vi "Example Program.vi"() -> ()   [LabVIEW 2014]
uses:
  Type Definitions/UTILITY Power Analyzer.ctl
panel:
  out "Average Power (Watts)":dbl format="%.3f"
  out "Output File":string[][](array[string])
  in  "Power Analyzer":T1
  in  "File Path Control":path=path "C:/Users/220038920/Desktop/CVS Folder/NI-2010/Trunk/Utility/Standby Power/Standby Power Settings.csv"
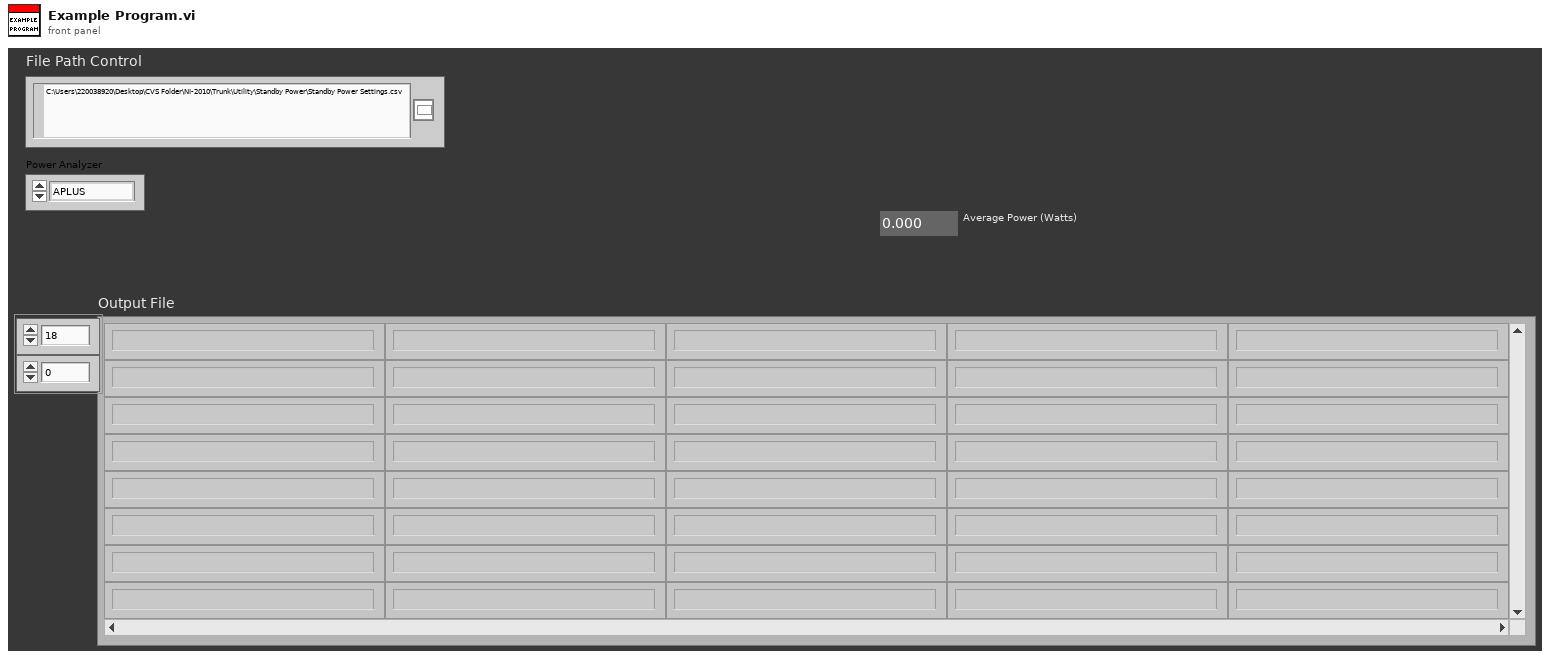
[diagram p1: front panel]
types:
  T1 = typedef "UTILITY Power Analyzer.ctl" = enum16{"APLUS", "WT210", "WT500", "WT300", "OSI", "Debug"}
  T2 = typedef "UTILITY Power Inputs Control.ctl" = cluster{"Yokogawa":cluster{"WT210":cluster{"Sample Rate (1: 0.25s)":i32, "A Range (12: 20A)":i32, "V Range (6: 600V)":i32, "Power VISA Yokogawa WT210":refnum<visa-resource-name>}, "WT500":cluster{"Power VISA Yokogawa WT500":refnum<visa-resource-name>, "V Range (8: 1000V)":i32, "I Range (7: 40A)":i32, "Update Rate (3: 500ms)":i32}}, "Aplus":cluster{"Aplus IP Address":string, "Remote Port":i32, "Instrument":string, "Instr Driver Revision":string}, "Power Limits":cluster{"Crest Factor":cluster{"Upper Limit":dbl, "Lower Limit":dbl}, "Harmonic Content":cluster{"Uthd":dbl}, "Voltage":cluster{"% Error":dbl}, "Stability":cluster{"<1 Watt ":cluster{"Wattage":dbl, "Slope (mW/H)":dbl}, ">1 Watt":cluster{"1%Power/Hour":dbl}}}, "Nominal Voltage":i32, "Time Limit (s)":dbl, "Power Variation Limit (%)":dbl, "Power Supply":cluster{"Chroma 61605":refnum<visa-resource-name>, "Use Chroma?":bool}}
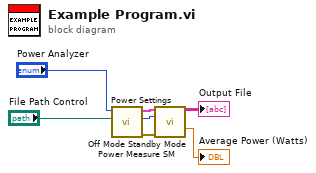
[diagram p0: block diagram]
diagram:
  n1 = call "Power Settings.vi"("File Path Control"="File Path Control", "Power Analyzer"="Power Analyzer") -> ("error out"=w3:errorcluster, "Power Analyzer Out"=w4:T1, "Power Out"=w7:T2)  [unwired: 7 in]
  n2 = call "Off Mode Standby Mode Power Measure SM.vi"("Power"=w7, "Power Analyzer"=w4, "Error In"=w3) -> ("Output File"=→"Output File":string[][], "Average Power (Watts)"=→"Average Power (Watts)":dbl)  [unwired: 8 in, 3 out]
